vi "Test Flatten.vi"() -> ()   [LabVIEW 2021]
uses:
  CIF_NIChn_FIFO_DAQ_DVR.lvclass
  CIFChannels/Typedef/Direction.ctl
  CIFChannels/CIFChannels.lvclass
  ChannelCommon/typedef/FIFO Header.ctl
  ChannelCommon/ChannelCommon.lvlib
  ChannelCommon/typedef/Datatype Waveform.ctl
  ChannelCommon/typedef/TimeStamps.ctl
panel:
  out "Pass":bool
  out "error out":errorcluster
  in  "FIFO Timestamps":T1={"ClockID"=2, "T0"=432, "T_Out"=543}
  out "Data out":T2[](array[typedef])=[{"measurement"=[0.0, 0.0, 0.0, 0.0, 0.0, 0.0, 0.0, 3.14], "dT"=0.01, "Timestamp"=498, "Read Lock"=FALSE}, {"measurement"=[0.0, 0.0, 0.0, 0.0, 0.0, 0.0, 0.0, 9.8], "dT"=0.12, "Timestamp"=12345, "Read Lock"=FALSE}]
  in  "Data In":T2[](array[typedef])=[{"measurement"=[0.0, 0.0, 0.0, 0.0, 0.0, 0.0, 0.0, 3.14], "dT"=0.01, "Timestamp"=498, "Read Lock"=FALSE}, {"measurement"=[0.0, 0.0, 0.0, 0.0, 0.0, 0.0, 0.0, 9.8], "dT"=0.12, "Timestamp"=12345, "Read Lock"=FALSE}]
  out "Header":T3={"Length"=57, "T0"=432, "T_Out"=543, "T_Tx"=1727639110950812000, "Ctr"=1, "ClockID"=2}
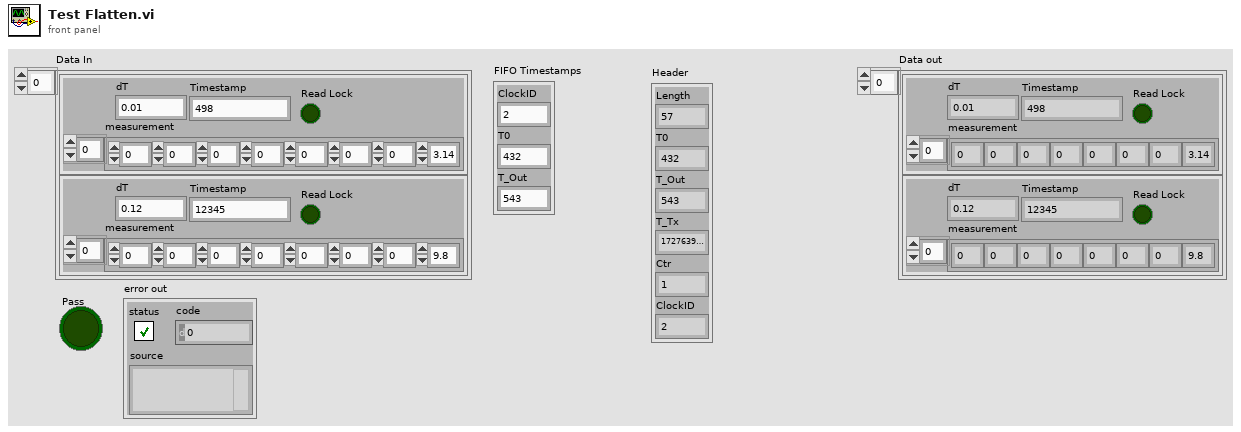
[diagram p1: front panel]
types:
  T1 = typedef "ChannelCommon.lvlib/TimeStamps.ctl" = cluster{"ClockID":u8, "T0":i64, "T_Out":i64}
  T2 = typedef "ChannelCommon.lvlib/Datatype Waveform.ctl" = cluster{"measurement":dbl[], "dT":dbl, "Timestamp":i64, "Read Lock":bool}
  T3 = typedef "ChannelCommon.lvlib/FIFO Header.ctl" = cluster{"Length":u64, "T0":i64, "T_Out":i64, "T_Tx":i64, "Ctr":u64, "ClockID":u8}
  T4 = typedef "CIFChannels.lvclass/Direction.ctl" = enum16{"Publisher", "Subscriber"}
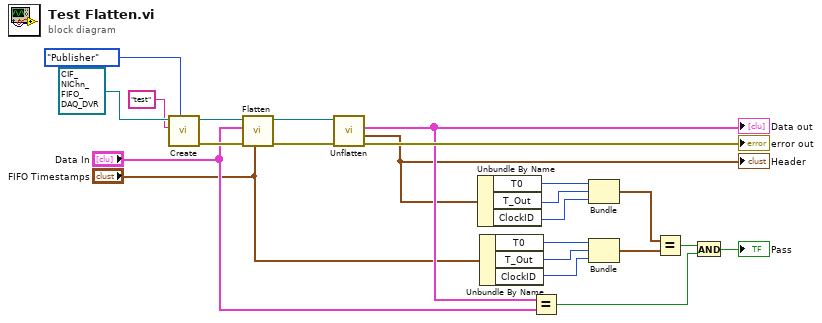
[diagram p0: block diagram]
diagram:
  n1 = call-dynamic "Create.vi"("Direction"=Direction."Publisher", "Name"="test", "CIF_NIChn_FIFO_DAQ in"=refnum<class "CIF_NIChn_FIFO_DAQ_DVR.lvclass"> refnum ("CIF_NIChn_Fifo_Power.lvclass")) -> ("error out"=w17:errorcluster, "CIF_NIChn_FIFO_DAQ out"=w19:refnum<class "CIF_NIChn_FIFO_DAQ_DVR.lvclass">)  [unwired: 7 in]
  n2 = call "Flatten.vi"("FIFO Timestamps"="FIFO Timestamps", "error in (no error)"=w17, "Data In"="Data In", "CIF_NIChn_FIFO_DAQ in"=w19) -> ("error out"=w18:errorcluster, "CIF_NIChn_FIFO_DAQ out"=w23:refnum<class "CIF_NIChn_FIFO_DAQ_DVR.lvclass">)  [unwired: 3 in, 3 out]
  n3 = call "Unflatten.vi"("error in (no error)"=w18, "CIF_NIChn_FIFO_DAQ in"=w23) -> ("error out"=→"error out":errorcluster, "Header"=w13:T3, "DAQ Out"=w15:T2[])  [unwired: 6 in, 1 out]
  "Header" <- w13
  "Data out" <- w15
  n4 = Unbundle By Name(w13) -> ("T0"=w11:i64, "T_Out"=w10:i64, "ClockID"=w9:u8)
  n5 = Unbundle By Name("FIFO Timestamps") -> ("T0"=w8:i64, "T_Out"=w7:i64, "ClockID"=w6:u8)
  n6 = Equal?(x=w15, y="Data In") -> (x = y?=w2:bool)
  n7 = Bundle("T0"=w11, "T_Out"=w10, "ClockID"=w9) -> (w4:cluster{"T0":i64, "T_Out":i64, "ClockID":u8})  [unwired: 1 in]
  n8 = Bundle("T0"=w8, "T_Out"=w7, "ClockID"=w6) -> (w5:cluster{"T0":i64, "T_Out":i64, "ClockID":u8})  [unwired: 1 in]
  n9 = Equal?(x=w4, y=w5) -> (x = y?=w3:bool)
  n10 = And(x=w3, y=w2) -> (x .and. y?=→"Pass":bool)
